vi "Mindsensors Pressure Sensor Config.vi"(10 "Node Data":T1, 11 "NXT":T2) -> ()   [LabVIEW 2010]
uses:
  <vilib>/NXT/Subs/LVHSConnector.ctl
  Datatypes/Node.ctl
  UI Controls/PlugInControls/Pluginbackground.ctl
  <vilib>/Utility/miscctls.llb/LVPointTypeDef.ctl
  <vilib>/NXT/Block Support/HWPage.SensorMode.ctl
  <vilib>/NXT/Block Support/HWPage.SensorType.ctl
  ConvertNodeAddrSensor.vi
panel:
  in  "Device Addr":i32 format="%.0x"
  out "Pressure":u16(graph)
  in  "Units":u16(ring) items=["PSI", "Millibar", "kPa"]
  out "?":dbl format="%#.2g"
  out "number":i8
  in  "Device Address":string
  in  "NXT Port":string
  in  "Name":string
  out "Headline":string="Type (auto populated)"
  in  "Sensor Parameters":string
  in  "Instance Specific Data":cluster{"Example Data":dbl}
  in  "Reset":bool
  in  "Save":bool
  in  "Stop":bool
  out "Background":T3=TRUE
  # "<- No controls below this line"
  # "Common controls such as Buttons, Rings, Sliders, Graphs, Decorations, etc can be found in the <labview>\\Targets\\NI\\NXT\\NXT Toolkit\\Schematic Editor\\UI Controls\\Plugin Controls\\ folder. Use these controls when possible to ensure a consistent look and feel with LabVIEW Education Edition."
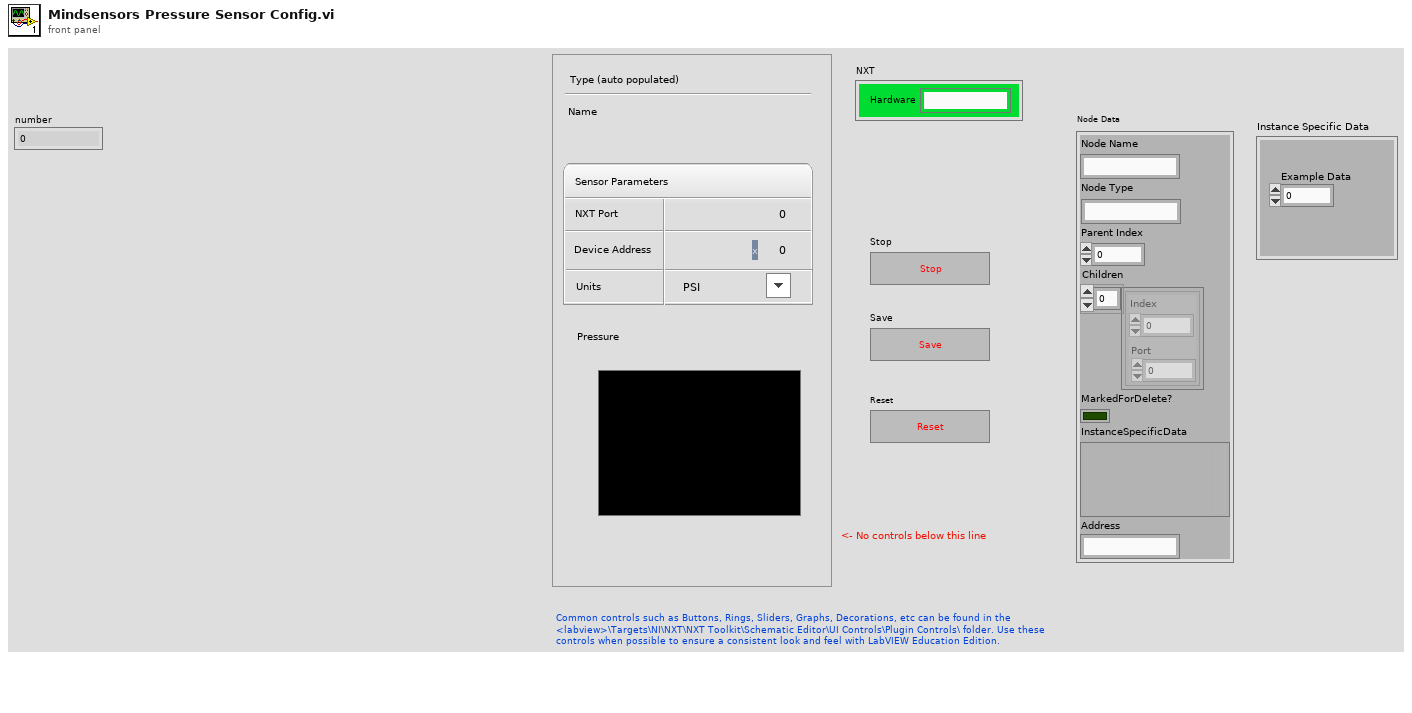
[diagram p1: front panel]
types:
  T1 = typedef "Node.ctl" = cluster{"Node Name":string, "Node Type":string, "Parent Index":i16, "Children":cluster{"Index":u16, "Port":u16}[], "MarkedForDelete?":bool, "InstanceSpecificData":variant, "Address":string}
  T2 = typedef "LVHSConnector.ctl" = cluster{"Hardware":string, "Flattened String":string}
  T3 = typedef "Pluginbackground.ctl" = bool
  T4 = typedef "LVPointTypeDef.ctl" = cluster{"Horizontal":i16, "Vertical":i16}
  T5 = enum8{"Enabled", "Disabled", "Disabled and Grayed Out"}
  T6 = typedef "HWPage.SensorMode.ctl" = u8
  T7 = typedef "HWPage.SensorType.ctl" = u8
  T8 = typedef "NXT_InputPort.ctl" = u8
  T9 = typedef "nxt.ctl" = cluster{"nxtHandle":u32, "fileHandle":u32, "fileIterHandle":u32, "moduleHandle":u32, "modIterHandle":u32, "nxtIterHandle":u32}
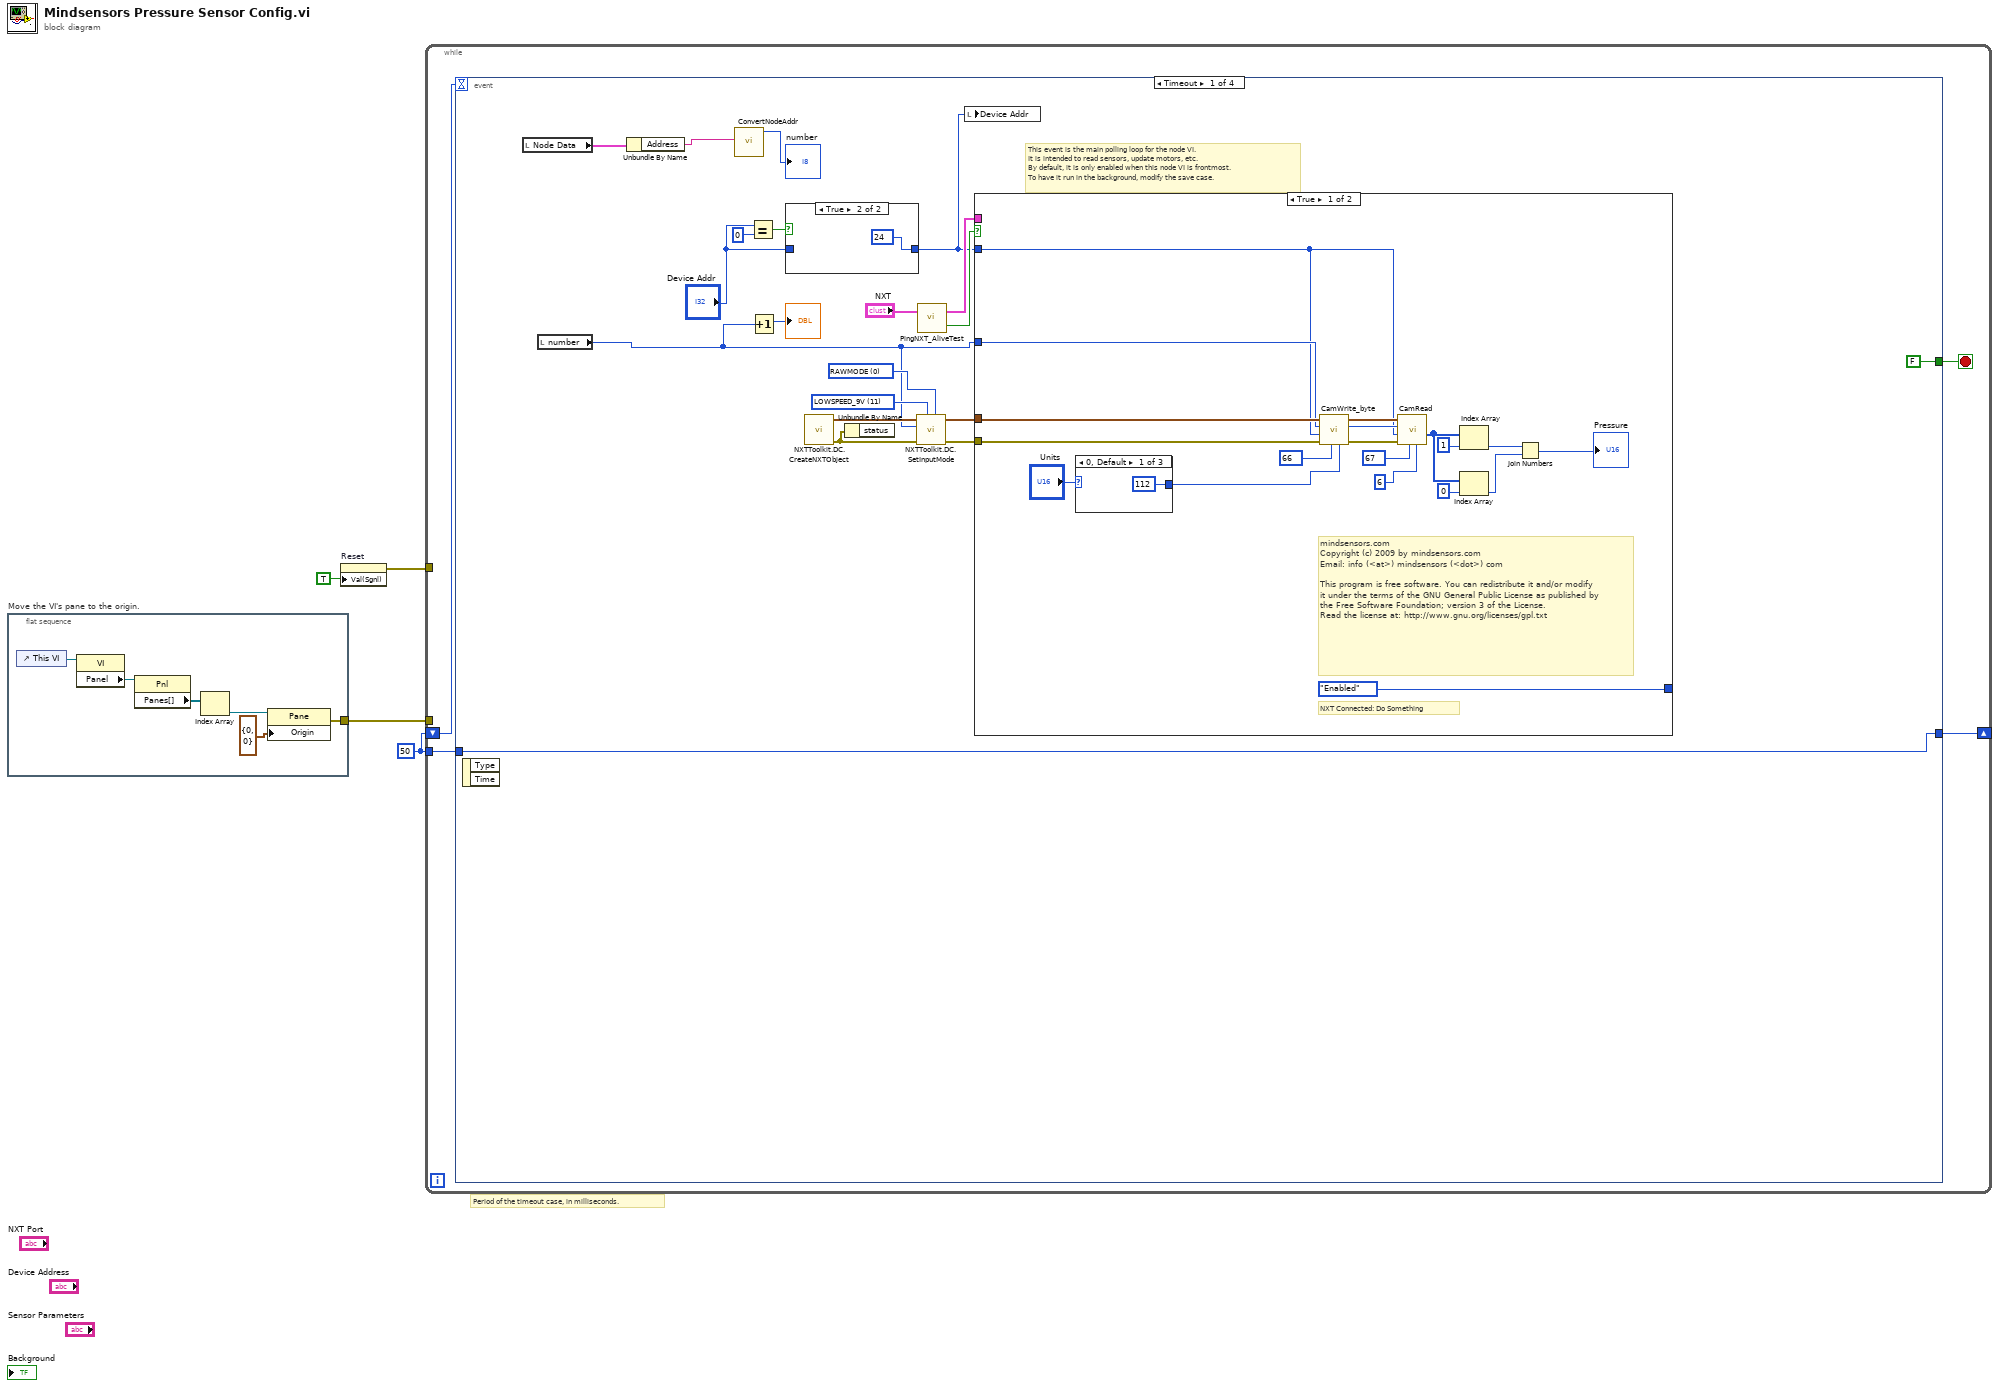
[diagram p0: block diagram]
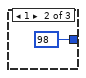
[diagram p3: hidden frame]
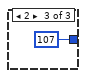
[diagram p4: hidden frame]
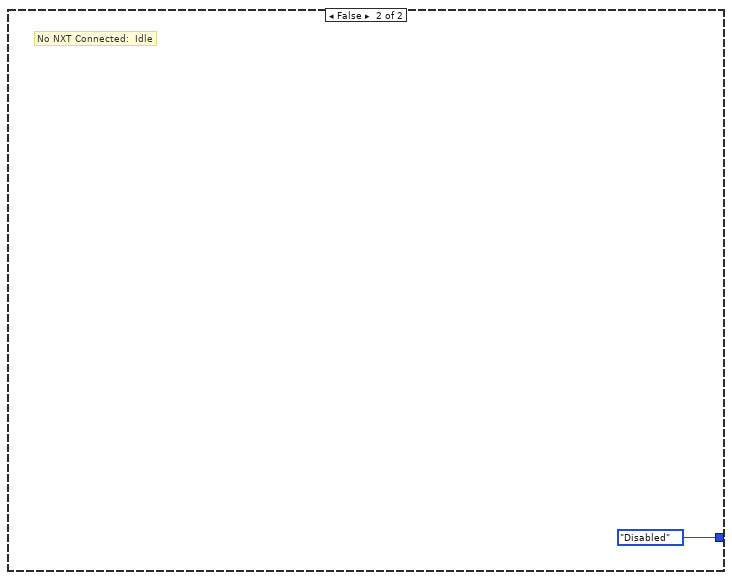
[diagram p5: hidden frame]
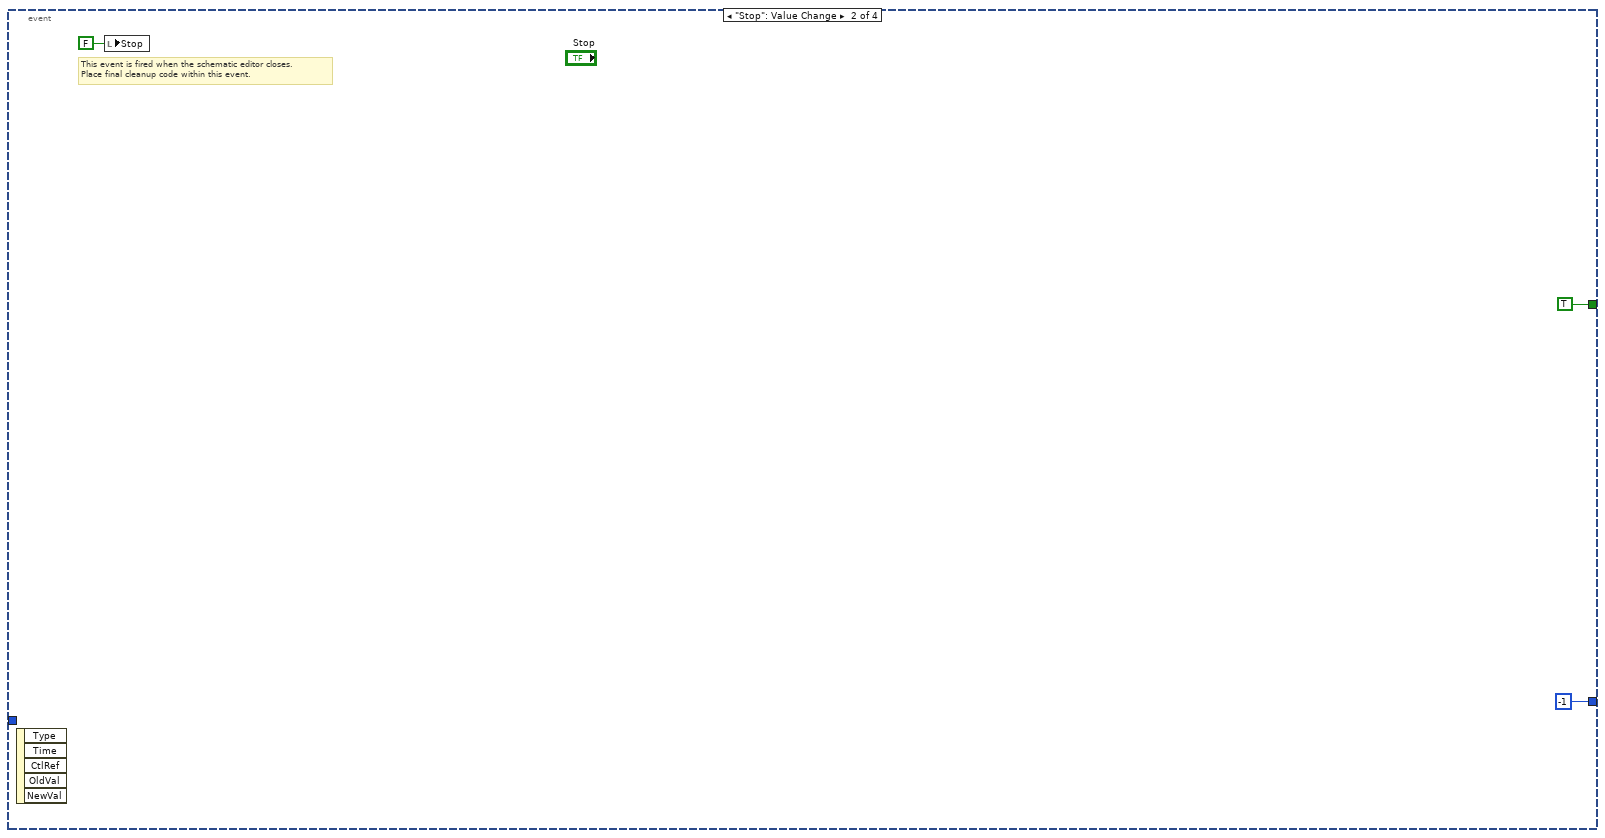
[diagram p6: hidden frame]
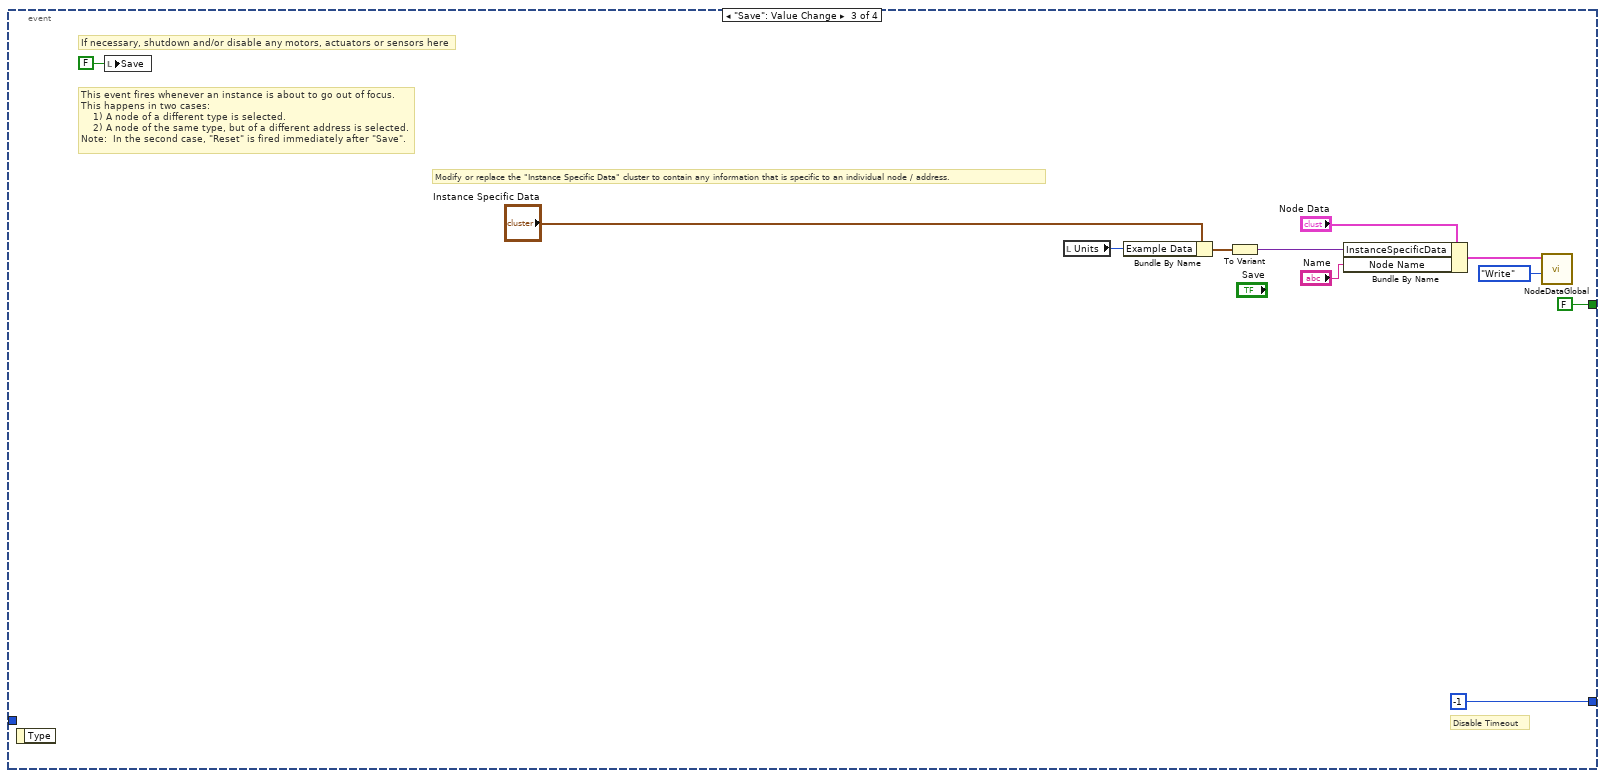
[diagram p7: hidden frame]
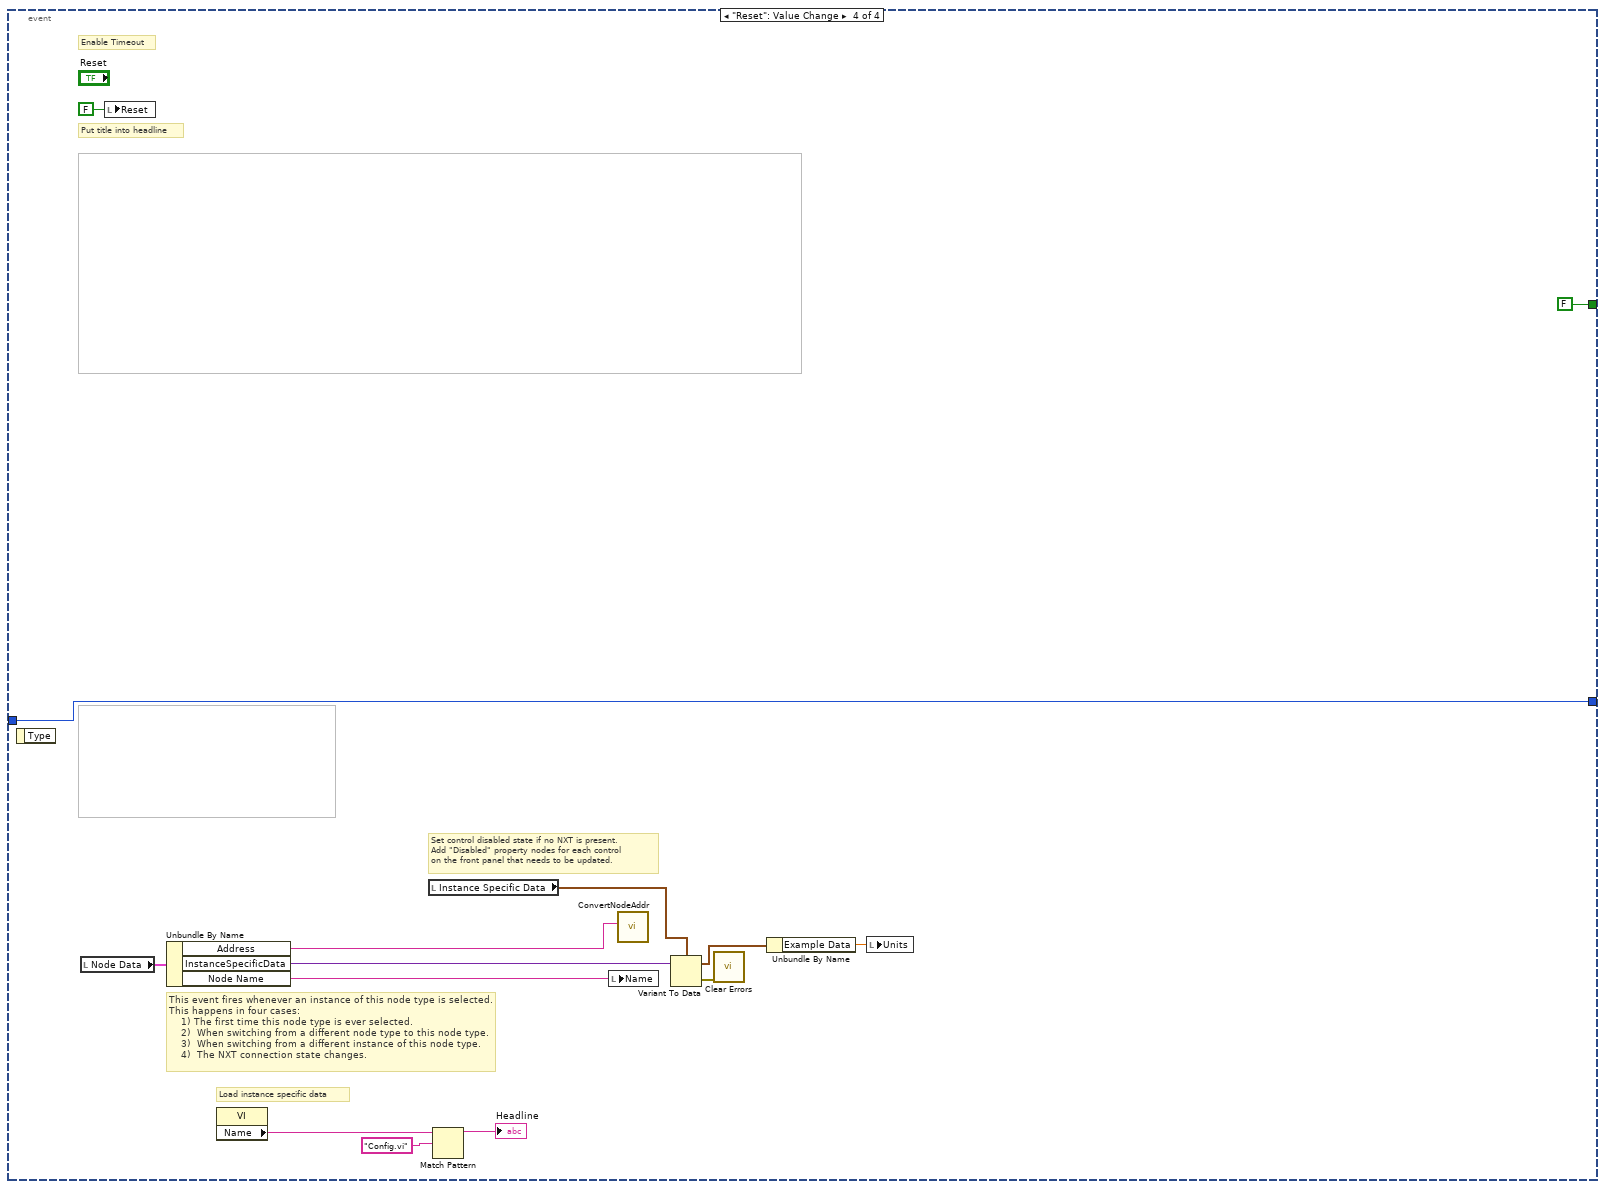
[diagram p8: hidden frame]
diagram:
  w2 = 50
  # "Period of the timeout case, in milliseconds."
  n1 = flat-sequence "Move the VI's pane to the origin." {
    tunnel: [w5] -> w1
    frame #0 {
      n2 = control-ref of="This VI"() -> (w6:refnum<vi>)
      n3 = property class="VI"(reference=w6) -> ("Panel"=w7:refnum<vi>)  [unwired: 1 in, 2 out]
      n4 = property class="Pnl"(reference=w7) -> ("Panes[]"=w8:refnum<vi>[])  [unwired: 1 in, 2 out]
      n5 = Index Array(array=w8) -> (element=w9:refnum<vi>)  [unwired: 1 in]
      n6 = property class="Pane"(reference=w9, "Origin"=T4 {"Horizontal"=0, "Vertical"=0}) -> (error out=w5:errorcluster)  [unwired: 1 in, 1 out]
    }
  }
  n7 = property on="Reset" class="Bool (strict)"("Val(Sgnl)"=TRUE ("Value (Signaling)")) -> (error out=w3:errorcluster)  [unwired: 2 in, 1 out]
  n8 = while {
    tunnel: w3 -> [_]
    shift-right: [w12] -> _
    shift-left: w2 -> [w13]
    tunnel: w2 -> [w11]
    tunnel: w1 -> [_]
    stop <- w14 stop-if-true
    n9 = event shown="[0] Timeout" {
      selector: _ -> [_ _ _ _]
      dyn-events: _ -> [_ _ _ _]
      timeout: w13 -> [_ _ _ _]
      tunnel: [FALSE TRUE FALSE FALSE] -> w14
      tunnel: [w33 -1 -1 w83] -> w12
      tunnel: w11 -> [w33 _ _ w83]
      event Timeout {
        w28 = T6 0 items=["RAWMODE"=0, "BOOLEANMODE"=32, "TRANSITIONCNTMODE"=64, "PERIODCOUNTERMODE"=96, "PCTFULLSCALEMODE"=128, "CELSIUSMODE"=160, "FAHRENHEITMODE"=192, "ANGLESTEPMODE"=224] ("Sensor Mode (RAWMODE)")
        w27 = T7 11 items=["NO_SENSOR", "SWITCH", "TEMPERATURE", "REFLECTION", "ANGLE", "LIGHT_ACTIVE", "LIGHT_INACTIVE", "SOUND_DB", "SOUND_DBA", "CUSTOM", "LOWSPEED", "LOWSPEED_9V", "HIGHSPEED"] ("Sensor Type (NO_SENSOR)")
        # "This event is the main polling loop for the node VI.\nIt is intended to read sensors, update motors, etc.\nBy default, it is only enabled when this node VI is frontmost.\nTo have it run in the background, modify the save case."
        n10 = event-data() -> ()  [unwired: 1 in, 2 out]
        n11 = local read "Node Data"() -> (w31:T1)
        n12 = local read "number"() -> (w16:i8)
        n13 = Unbundle By Name(w31) -> ("Address"=w18:string)
        n14 = call-poly "ConvertNodeAddr.vi"("Sensor Port"=w18) -> ("NXT Port"=→"number":T8)  [unwired: 6 in, 4 out]
        n15 = Equal?(x="Device Addr", y=u8 0) -> (x = y?=w21:bool)
        n16 = Increment(x=w16) -> (x+1=→"?":i8)
        n17 = case shown="True" w21 {
          tunnel: [w35 u8 24 ("Device Addr 2")] -> w20
          tunnel: "Device Addr" -> [w35 _]
          frame False {
          }
          frame True {
          }
        }
        n18 = call <vilib>:"NXTToolkit.DC.CreateNXTObject.vi"() -> ("error out"=w25:errorcluster, "NXTObject"=w26:T9)  [unwired: 9 in, 1 out]
        n19 = Unbundle By Name(w25) -> ()  [unwired: 1 out]
        n20 = call <vilib>:"NXTToolkit.DC.SetInputMode.vi"("Sensor Mode (RAWMODE)"=w28, "Sensor Type (NO_SENSOR)"=w27, "error in (no error)"=w25, "Input Port (Port 1)"=w16, "NXTObject"=w26) -> ("error out"=w23:errorcluster, "NXTObject dup"=w24:T9)  [unwired: 4 in, 1 out]
        n21 = call <vilib>:"PingNXT_AliveTest.vi"("NXT"="NXT") -> ("connected?"=w30:bool, "NXT"=w29:T2)  [unwired: 1 in]
        n22 = local write "Device Addr"(w20) -> ()
        n23 = case shown="True" w30 {
          tunnel: [T5."Enabled" ("Disabled") T5."Disabled" ("Disabled")] -> _
          tunnel: w29 -> [_ _]
          tunnel: w24 -> [w48 _]
          tunnel: w23 -> [w47 _]
          tunnel: w16 -> [w40 _]
          tunnel: w20 -> [w39 _]
          frame True {
            # "mindsensors.com\nCopyright (c) 2009 by mindsensors.com\nEmail: info (<at>) mindsensors (<dot>) com\n\nThis program is free software. You can redistribute it and/or modify\nit under the terms of the GNU General Public License as published by\nthe Free Software Foundation; version 3 of the License.\nRead the license at: http://www.gnu.org/licenses/gpl.txt"
            # "NXT Connected: Do Something"
            n24 = case shown="0, Default" "Units" {
              tunnel: [112 98 107] -> w37
              frame 0, Default {
              }
              frame 1 {
              }
              frame 2 {
              }
            }
            n25 = call <vilib>:"CamWrite_byte.vi"("Data byte"=w37, "Reg Address"=u8 66, "error in (no error)"=w47, "Device Address"=w39, "Input Port in"=w40, "NXTObject"=w48) -> ("error out"=w41:errorcluster, "Input Port dup"=w42:T8, "NXTObject dup"=w43:T9)  [unwired: 1 in, 2 out]
            n26 = call <vilib>:"CamRead.vi"("bytes to read"=u8 6, "Reg Address"=u8 67, "error in (no error)"=w41, "Device Address"=w39, "Input Port in"=w42, "NXTObject"=w43) -> ("data Buffer"=w52:u8[])  [unwired: 5 out]
            n27 = Index Array(array=w52, index=1) -> (element=w49:u8)
            n28 = Index Array(array=w52, index=0) -> (element=w50:u8)
            n29 = Join Numbers(hi=w49, lo=w50) -> ((hi.lo)=→"Pressure":u16)
          }
          frame False {
            # "No NXT Connected:  Idle"
          }
        }
      }
      event "Stop": Value Change {
        # "This event is fired when the schematic editor closes.\nPlace final cleanup code within this event."
        n30 = event-data() -> ()  [unwired: 1 in, 5 out]
        n31 = local write "Stop"(FALSE ("stop")) -> ()
      }
      event "Save": Value Change {
        # "If necessary, shutdown and/or disable any motors, actuators or sensors here"
        # "Modify or replace the \"Instance Specific Data\" cluster to contain any information that is specific to an individual node / address."
        # "Disable Timeout"
        # "This event fires whenever an instance is about to go out of focus.\nThis happens in two cases:\n    1) A node of a different type is selected.\n    2) A node of the same type, but of a different address is selected.\nNote:  In the second case, \"Reset\" is fired immediately after \"Save\"."
        n32 = event-data() -> ()  [unwired: 1 in, 1 out]
        n33 = local write "Save"(FALSE ("stop")) -> ()
        n34 = local read "Units"() -> (w63:u16)
        n35 = Bundle By Name(cluster="Instance Specific Data", "Example Data"=w63) -> (w64:cluster{"Example Data":dbl})
        n36 = To Variant(anything=w64) -> (Variant=w71:variant)
        n37 = Bundle By Name(cluster="Node Data", "InstanceSpecificData"=w71, "Node Name"="Name") -> (w70:T1)
        n38 = call "NodeDataGlobal.vi"("Action"=enum16{"Read", "Write"}."Write", "Node Data In"=w70) -> ()  [unwired: 8 in, 2 out]
      }
      event "Reset": Value Change {
        # "Set control disabled state if no NXT is present.\nAdd \"Disabled\" property nodes for each control\non the front panel that needs to be updated."
        # "Load instance specific data"
        # "Enable Timeout"
        # "This event fires whenever an instance of this node type is selected.\nThis happens in four cases:\n    1) The first time this node type is ever selected.\n    2)  When switching from a different node type to this node type.\n    3)  When switching from a different instance of this node type. \n    4)  The NXT connection state changes."
        # "Put title into headline"
        n39 = event-data() -> ()  [unwired: 1 in, 1 out]
        n40 = local read "Node Data"() -> (w84:T1)
        n41 = local write "Reset"(FALSE ("Reset")) -> ()
        n42 = Unbundle By Name(w84) -> ("Address"=w75:string, "InstanceSpecificData"=w85:variant, "Node Name"=w77:string)
        n43 = property class="VI"() -> ("Name"=w79:string)  [unwired: 2 in, 2 out]
        n44 = local read "Instance Specific Data"() -> (w82:cluster{"Example Data":dbl})
        n45 = Match Pattern(string=w79, regular expression="Config.vi") -> (before substring=→"Headline":string)  [unwired: 1 in, 3 out]
        n46 = local write "Name"(w77) -> ()
        n47 = call-poly "ConvertNodeAddr.vi"("Sensor Port"=w75) -> ()  [unwired: 6 in, 5 out]
        n48 = Variant To Data(Variant=w85, type=w82) -> (error out=w81:errorcluster, data=w76:cluster{"Example Data":dbl})  [unwired: 1 in]
        n49 = call <vilib>:"Clear Errors.vi"("error in (no error)"=w81) -> ()  [unwired: 6 in, 1 out]
        n50 = Unbundle By Name(w76) -> ("Example Data"=w74:dbl)
        n51 = local write "Units"(w74) -> ()
      }
    }
  }
